vi "Create (I16 Array).vi"(6 "timestamp in":timestamp, 7 "fields":T1, 8 "error in (no error)":errorcluster, 10 "value in":i16[](array[numeric])) -> (0 "error out":errorcluster, 2 "value out":i16[](array[numeric]), 3 "NT Scalar (Numeric) out":refnum<class "NT Scalar (Numeric).lvclass">, 4 "timestamp out":timestamp)   [LabVIEW 2020, in "PV Access.lvlib" / "PV Data.lvlib" / "NT Scalar (Numeric).lvclass"]
uses:
  NT Scalar (Numeric).lvclass
  C:/Users/eyw68381/source/repos/pvaccess-labview/labview/source/PV Data/NT Base/NT Base.lvclass
  Value Fields.ctl
  PV Data.lvlib
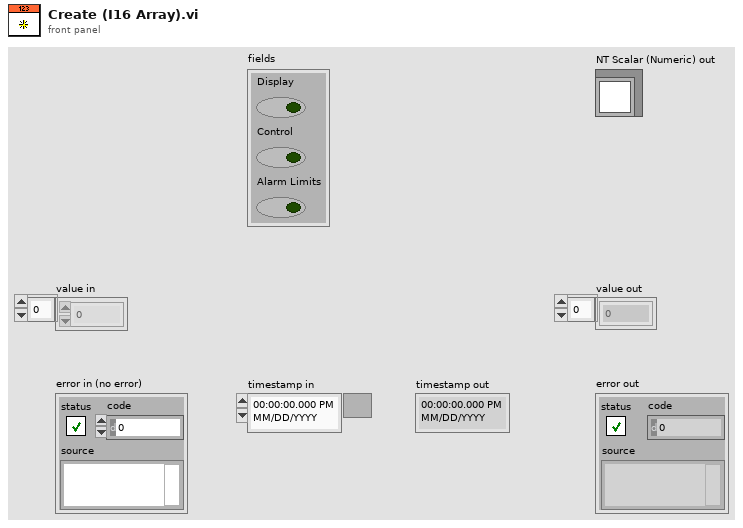
[diagram p1: front panel]
types:
  T1 = typedef "PV Access.lvlib/PV Data.lvlib/Value Fields.ctl" = cluster{"Display":bool, "Control":bool, "Alarm Limits":bool}
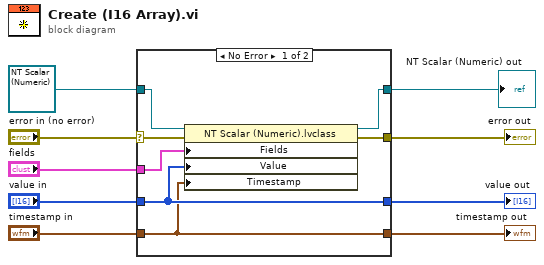
[diagram p0: block diagram]
diagram:
  n1 = case shown="No Error" "error in (no error)" {
    selector: "error in (no error)" -> [w16 w20]
    tunnel: [w14 w20] -> w8
    tunnel: [w15 w19] -> w6
    tunnel: refnum<class "NT Scalar (Numeric).lvclass"> refnum ("NT Scalar (Numeric) in") -> [w13 w19]
    tunnel: "value in" -> [w11 w18]
    tunnel: [w11 w18] -> w5
    tunnel: "fields" -> [w12 _]
    tunnel: "timestamp in" -> [w10 w17]
    tunnel: [w10 w17] -> w1
    frame No Error {
      n2 = property class="NT Scalar (Numeric).lvclass"(reference=w13, error in=w16, "Fields"=w12, "Value"=w11, "Timestamp"=w10) -> (reference out=w15:refnum<class "NT Scalar (Numeric).lvclass">, error out=w14:errorcluster)
    }
    frame Error {
    }
  }
  "error out" <- w8
  "NT Scalar (Numeric) out" <- w6
  "value out" <- w5
  "timestamp out" <- w1
